vi "ConvertImageToQTFormat.vi"(1 "image data":T1) -> (0 "Image Out":T2 {"Dialogs" format="%.0b"})   [LabVIEW 2024]
uses:
  <userlib>/ImageProcessing/QTLIB_2595_LV86/QT_Image.ctl
  <vilib>/picture/picture.llb/imagedata.ctl
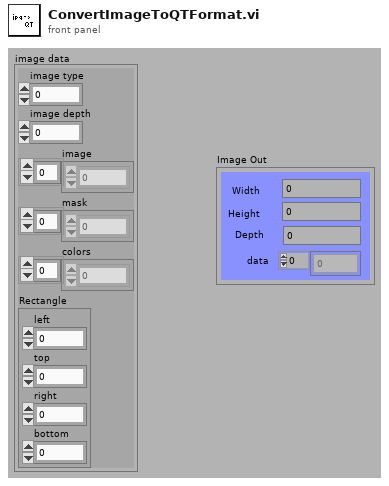
[diagram p1: front panel]
types:
  T1 = typedef "imagedata.ctl" = cluster{"image type":i32, "image depth":i32, "image":u8[], "mask":u8[], "colors":u32[], "Rectangle":cluster{"left":i16, "top":i16, "right":i16, "bottom":i16}}
  T2 = typedef "QT_Image.ctl" = cluster{"Width":i32, "Height":i32, "Depth":i32, "data":u8[], "Compressed data":u8[], "Color table":u32[], "Duration":i32, "Options":i32, "Timestamp":i32, "ID":i32, "Reserved":i32, "Dialogs":u32}
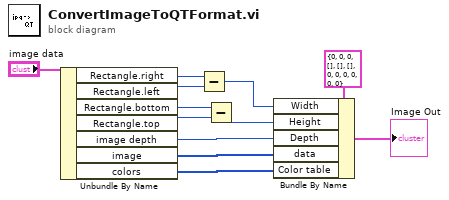
[diagram p0: block diagram]
diagram:
  n1 = Unbundle By Name("image data") -> ("Rectangle.right"=w6:i16, "Rectangle.left"=w5:i16, "Rectangle.bottom"=w9:i16, "Rectangle.top"=w8:i16, "image depth"=w3:i32, "image"=w2:u8[], "colors"=w1:u32[])
  n2 = Subtract(x=w6, y=w5) -> (x-y=w4:i16)
  n3 = Subtract(x=w9, y=w8) -> (x-y=w7:i16)
  n4 = Bundle By Name(cluster=T2 {"Width"=0, "Height"=0, "Depth"=0, "data"=[], "Compressed data"=[], "Color table"=[], "Duration"=0, "Options"=0, "Timestamp"=0, "ID"=0, "Reserved"=0, "Dialogs"=0} ("Image Out"), "Width"=w4, "Height"=w7, "Depth"=w3, "data"=w2, "Color table"=w1) -> (→"Image Out":T2)
